vi "Create All Message Queues.vi"(8 "error in (no error)":errorcluster) -> (0 "error out":errorcluster, 3 "Message Queues out":T1)   [LabVIEW 2019, in "Message Queue.lvlib"]
doc: "This VI creates and initializes all the message queues for your application. If your application requires more than one message queue, right-click the \"Message Queues\" constant above and select Open Type Def. Add the new Message Queue(s) to the type definition, then initialize them in this VI."
uses:
  Message Queue.lvlib
  All Message Queues.ctl
  Message Cluster.ctl
  Enqueue Message (Single).vi
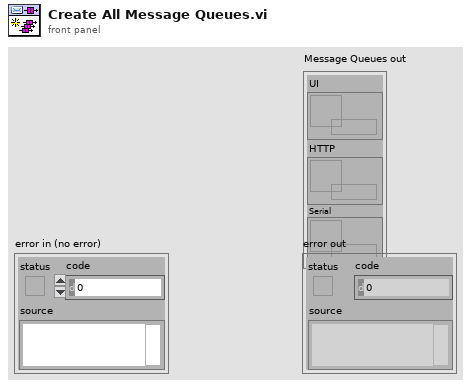
[diagram p1: front panel]
types:
  T1 = typedef "Message Queue.lvlib/All Message Queues.ctl" = cluster{"UI":refnum<queue>, "HTTP":refnum<queue>, "Serial":refnum<queue>}
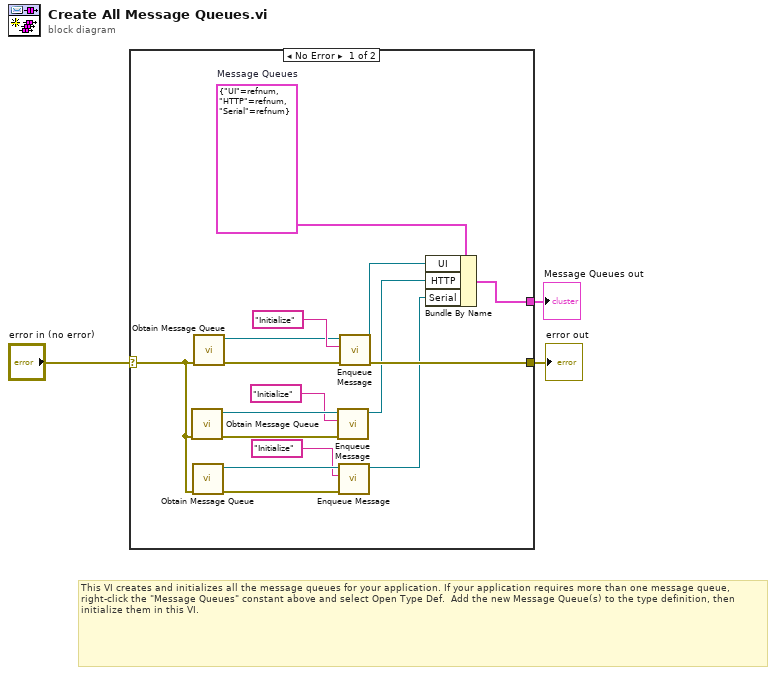
[diagram p0: block diagram]
diagram:
  # "This VI creates and initializes all the message queues for your application. If your application requires more than one message queue, right-click the \"Message Queues\" constant above and select Open Type Def.  Add the new Message Queue(s) to the type definition, then initialize them in this VI."
  n1 = case shown="No Error" "error in (no error)" {
    selector: "error in (no error)" -> [w6 w20]
    tunnel: [w19 w20] -> w3
    tunnel: [w17 _] -> w2
    frame No Error {
      w18 = T1 {"UI"=refnum, "HTTP"=refnum, "Serial"=refnum}  # Message Queues
      n2 = call "Obtain Message Queue.vi"("error in (no error)"=w6) -> ("error out"=w11:errorcluster, "Message Queue"=w13:refnum<queue>)  [unwired: 9 in]
      n3 = call "Obtain Message Queue.vi"("error in (no error)"=w6) -> ("error out"=w8:errorcluster, "Message Queue"=w7:refnum<queue>)  [unwired: 9 in]
      n4 = call "Obtain Message Queue.vi"("error in (no error)"=w6) -> ("error out"=w16:errorcluster, "Message Queue"=w14:refnum<queue>)  [unwired: 9 in]
      n5 = call-poly "Enqueue Message.vi"("error in (no error)"=w11, "Message"="Initialize", "Message Queue"=w13) -> ("dup Message Queue"=w10:refnum<queue>)  [unwired: 7 in, 1 out]
      n6 = call-poly "Enqueue Message.vi"("error in (no error)"=w8, "Message"="Initialize", "Message Queue"=w7) -> ("dup Message Queue"=w5:refnum<queue>)  [unwired: 7 in, 1 out]
      n7 = call-poly "Enqueue Message.vi"("error in (no error)"=w16, "Message"="Initialize", "Message Queue"=w14) -> ("error out"=w19:errorcluster, "dup Message Queue"=w9:refnum<queue>)  [unwired: 7 in]
      n8 = Bundle By Name(cluster=w18, "UI"=w9, "HTTP"=w10, "Serial"=w5) -> (w17:T1)
    }
    frame Error {
    }
  }
  "Message Queues out" <- w2
  "error out" <- w3
